vi "Read topicClusterCtrlRefRef.vi"(11 "PolymorphicInstance in":refnum<class "PolymorphicInstance.lvclass">) -> (2 "topicClusterCtrlRefRef":refnum<vi>, 3 "PolymorphicInstance out":refnum<class "PolymorphicInstance.lvclass">)   [LabVIEW 2012, in "PolymorphicInstance.lvclass"]
uses:
  PolymorphicInstance.lvclass
  PolymorphicInstance.lvclass/PolymorphicInstance.ctl
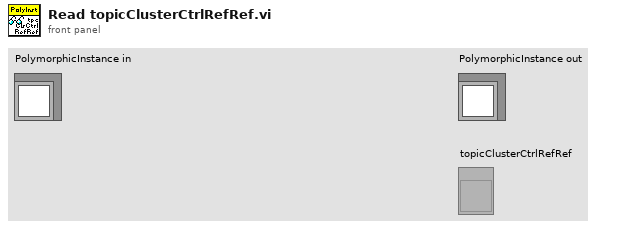
[diagram p1: front panel]
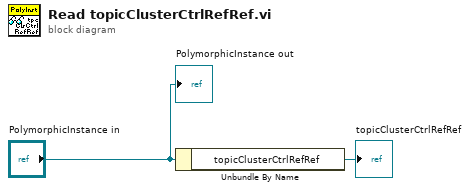
[diagram p0: block diagram]
diagram:
  n1 = Unbundle By Name("PolymorphicInstance in") -> ("topicClusterCtrlRefRef"=→"topicClusterCtrlRefRef":refnum<vi>)
  "PolymorphicInstance out" <- "PolymorphicInstance in"
